vi "sine and cosine using bundle.vi"() -> ()   [LabVIEW 2020]
panel:
  in  "stop":bool
  out "Waveform Chart":cluster{dbl, dbl}(graph)
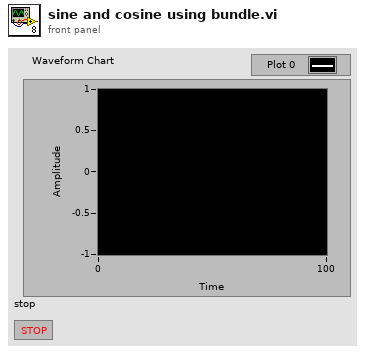
[diagram p1: front panel]
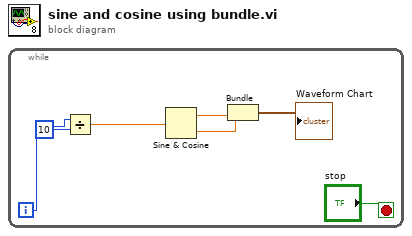
[diagram p0: block diagram]
diagram:
  n1 = while {
    i -> [w5]
    stop <- "stop" stop-if-true
    n2 = Divide(x=w5, y=10) -> (x/y=w6:dbl)
    n3 = Sine & Cosine(0:w6) -> (1:w1:dbl, 2:w3:dbl)
    n4 = Bundle(w3, w1) -> (→"Waveform Chart":cluster{dbl, dbl})  [unwired: 1 in]
  }
